vi "Init Data.vi"(10 "Data":T1) -> (3 "Msg out":refnum<class "Msg.lvclass">)   [LabVIEW 2020, in "BoolData.lvlib" / "Msg.lvclass"]
uses:
  Msg.lvclass
  Data.ctl
  Msg.lvclass/Msg.ctl
  BoolData.lvlib
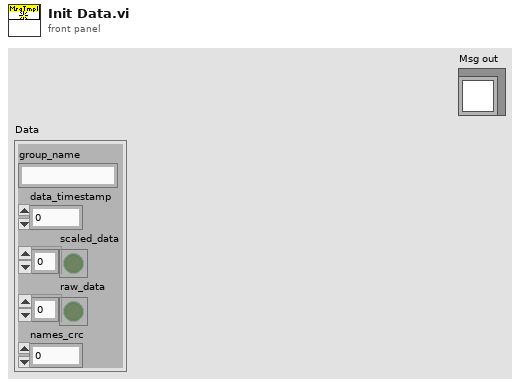
[diagram p1: front panel]
types:
  T1 = typedef "BoolData.lvlib/Data.ctl" = cluster{"group_name":string, "data_timestamp":i64, "scaled_data":bool[], "raw_data":bool[], "names_crc":u32}
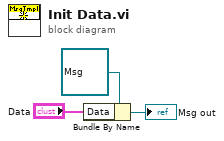
[diagram p0: block diagram]
diagram:
  n1 = Bundle By Name(cluster=refnum<class "Msg.lvclass"> refnum ("Msg out"), "Data"="Data") -> (→"Msg out":refnum<class "Msg.lvclass">)
